vi "GetProperties.vi"(8 "error in":errorcluster, 11 "Array in":refnum<class "Array.lvclass">) -> (0 "error out":errorcluster, 3 "Array out":refnum<class "Array.lvclass">)   [LabVIEW 2014, in "Array.lvclass"]
uses:
  Array.lvclass
  Array.lvclass/Array.ctl
  Control/Control.lvclass
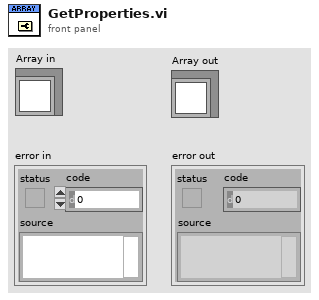
[diagram p1: front panel]
types:
  T1 = typedef "LVRectTypeDef.ctl" = cluster{"Left":i16, "Top":i16, "Right":i16, "Bottom":i16}
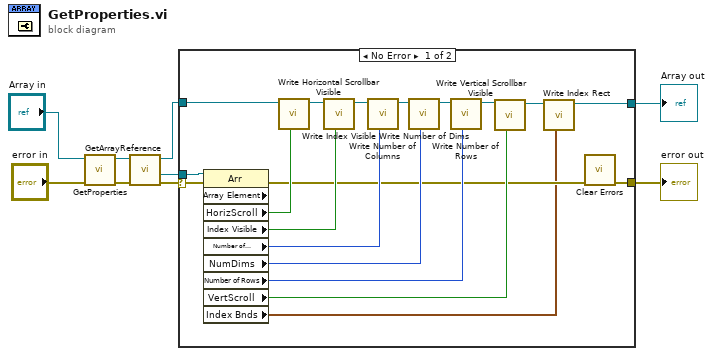
[diagram p0: block diagram]
diagram:
  n1 = call-parent "GetProperties.vi"("error in"="error in", "Control in"="Array in") -> ("error out"=w6:errorcluster, "Control out"=w7:refnum<class "Array.lvclass">)  [unwired: 8 in]
  n2 = call "GetArrayReference.vi"("error in"=w6, "Array in"=w7) -> ("error out"=w5:errorcluster, "array reference"=w4:refnum<vi>, "Array out"=w3:refnum<class "Array.lvclass">)  [unwired: 7 in]
  n3 = case shown="No Error" w5 {
    selector: w5 -> [w28 w29]
    tunnel: w4 -> [w27 _]
    tunnel: w3 -> [w14 w30]
    tunnel: [w10 w29] -> w1
    tunnel: [w12 w30] -> w2
    frame No Error {
      n4 = property class="Arr" props=["Array Element", "HorizScroll", "Index Visible", "Number of Columns", "NumDims", "Number of Rows", "VertScroll", "Index Bnds"](reference=w27, error in=w28) -> (error out=w15:errorcluster, "HorizScroll"=w26:bool, "Index Visible"=w24:bool, "Number of Columns"=w22:u32, "NumDims"=w20:u32, "Number of Rows"=w18:u32, "VertScroll"=w16:bool, "Index Bnds"=w11:T1)  [unwired: 2 out]
      n5 = call "Write Horizontal Scrollbar Visible.vi"("Horizontal Scrollbar Visible"=w26, "Array in"=w14) -> ("Array out"=w25:refnum<class "Array.lvclass">)  [unwired: 7 in]
      n6 = call "Write Index Visible.vi"("Index Visible"=w24, "Array in"=w25) -> ("Array out"=w23:refnum<class "Array.lvclass">)  [unwired: 7 in]
      n7 = call "Write Number of Columns.vi"("Number of Columns"=w22, "Array in"=w23) -> ("Array out"=w21:refnum<class "Array.lvclass">)  [unwired: 7 in]
      n8 = call "Write Number of Dims.vi"("Number of Dims"=w20, "Array in"=w21) -> ("Array out"=w19:refnum<class "Array.lvclass">)  [unwired: 7 in]
      n9 = call "Write Number of Rows.vi"("Number of Rows"=w18, "Array in"=w19) -> ("Array out"=w17:refnum<class "Array.lvclass">)  [unwired: 7 in]
      n10 = call "Write Vertical Scrollbar Visible.vi"("Vertical Scrollbar Visible"=w16, "Array in"=w17) -> ("Array out"=w13:refnum<class "Array.lvclass">)  [unwired: 7 in]
      n11 = call "Write Index Rect.vi"("Index Rect"=w11, "Array in"=w13) -> ("Array out"=w12:refnum<class "Array.lvclass">)  [unwired: 7 in]
      n12 = call <vilib>:"Clear Errors.vi"("error in (no error)"=w15) -> ("error out"=w10:errorcluster)  [unwired: 5 in, 1 out]
    }
    frame Error {
    }
  }
  "error out" <- w1
  "Array out" <- w2
